vi "ImPro - Open Image.vi"(8 "error in (no error)":errorcluster, 11 "path to PNG file":path) -> (0 "error out":errorcluster, 1 "Rectangle":T1, 2 "24-bit pixmap":u32[][](array[numeric]), 3 "new picture":picture)   [LabVIEW 2023]
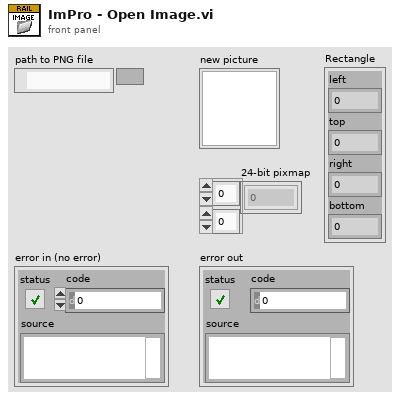
[diagram p1: front panel]
types:
  T1 = cluster{"left":i16, "top":i16, "right":i16, "bottom":i16}
  T2 = typedef "imagedata.ctl" = cluster{"image type":i32, "image depth":i32, "image":u8[], "mask":u8[], "colors":u32[], "Rectangle":cluster{"left":i16, "top":i16, "right":i16, "bottom":i16}}
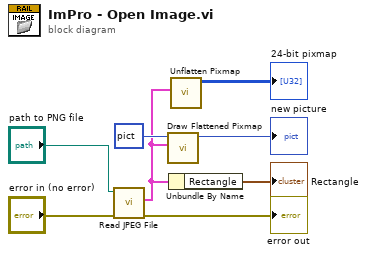
[diagram p0: block diagram]
diagram:
  n1 = call <vilib>:"Read JPEG File.vi"("error in (no error)"="error in (no error)", "path to JPEG file"="path to PNG file") -> ("error out"=→"error out":errorcluster, "image data"=w2:T2)  [unwired: 7 in, 1 out]
  n2 = call <vilib>:"Draw Flattened Pixmap.vi"("image data"=w2, "picture"=picture data[5B]) -> ("new picture"=→"new picture":picture)  [unwired: 7 in]
  n3 = Unbundle By Name(w2) -> ("Rectangle"=→"Rectangle":T1)
  n4 = call <vilib>:"Unflatten Pixmap.vi"("image data"=w2) -> ("24-bit pixmap"=→"24-bit pixmap":u32[][])  [unwired: 4 in, 6 out]
